vi "GetCodeTag.vi"(8 "error in (no error)":errorcluster, 11 "Code in":refnum<class "Code.lvclass">) -> (0 "error out":errorcluster, 2 "CodeTag":string, 3 "Code out":refnum<class "Code.lvclass">)   [LabVIEW 2021, in "Markdown.lvlib" / "Code.lvclass"]
uses:
  Code.lvclass
  Code.lvclass/Code.ctl
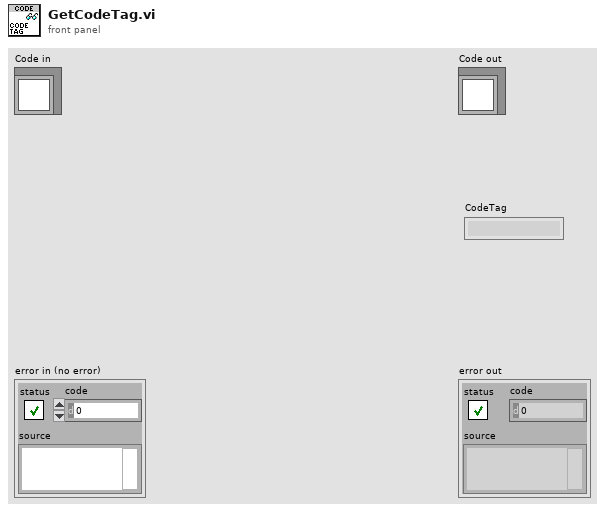
[diagram p1: front panel]
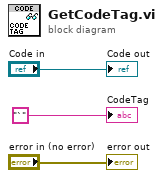
[diagram p0: block diagram]
diagram:
  "error out" <- "error in (no error)"
  "Code out" <- "Code in"
  "CodeTag" <- "`" ("BoldTag")
